vi "Filter Clusters.vi"(8 "Error In":errorcluster) -> (0 "Error Out":errorcluster)   [LabVIEW 2017]
uses:
  <vilib>/Utility/traverseref.llb/TRef TravTarget.ctl
  Support VIs/Filter Clusters Target.vi
  <vilib>/addons/_JKI Toolkits/Caraya/classes/Test/Test.lvclass
  Toolkit.lvlib
  <vilib>/Utility/traverseref.llb/VI Scripting - Traverse.lvlib
  src/Toolkit/Toolkit.lvlib
  <vilib>/addons/_JKI Toolkits/Caraya/classes/Assert/Assert.lvclass
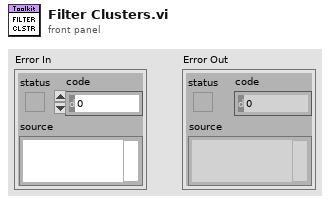
[diagram p1: front panel]
types:
  T1 = typedef "TRef TravTarget.ctl" = enum16{"FP", "BD", "Other"}
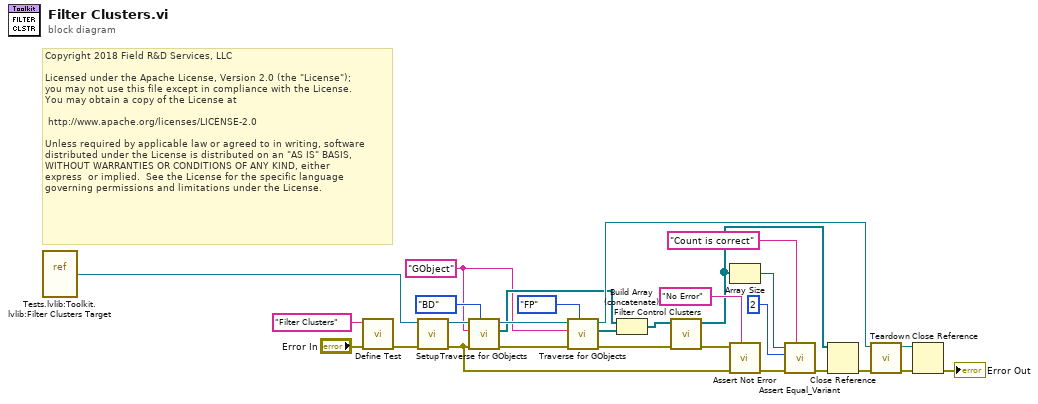
[diagram p0: block diagram]
diagram:
  w1 = "GObject" ("Class Name")
  # "Copyright 2018 Field R&D Services, LLC\n\nLicensed under the Apache License, Version 2.0 (the \"License\");\nyou may not use this file except in compliance with the License.\nYou may obtain a copy of the License at\n\n\thttp://www.apache.org/licenses/LICENSE-2.0\n\nUnless required by applicable law or agreed to in writing, software\ndistributed under the License is distributed on an \"AS IS\" BASIS,\nWITHOUT WARRANTIES OR CONDITIONS OF ANY KIND, either \nexpress  or implied.  See the License for the specific language \ngoverning permissions and limitations under the License."
  n1 = vi-ref "Tests.lvlib:Toolkit.lvlib:Filter Clusters Target.vi"() -> (w25:refnum<vi>)
  n2 = call <vilib>:"Define Test.vi"("error in (no error)"="Error In", "Label (VI Title)"="Filter Clusters") -> ("error out"=w26:errorcluster)  [unwired: 9 in]
  n3 = call "Setup.vi"("Error In"=w26, "VI In"=w25) -> ("Error Out"=w19:errorcluster, "VI Out"=w23:refnum<vi>)  [unwired: 8 in]
  n4 = call <vilib>:"Traverse for GObjects.vi"("Traverse Target"=TRef_TravTarget."BD", "error in (no error)"=w19, "Class Name"=w1, "VI Refnum"=w23) -> ("error out"=w8:errorcluster, "References"=w4:refnum<vi>[], "dup VI Refnum"=w9:refnum<vi>)  [unwired: 4 in, 1 out]
  n5 = call <vilib>:"Traverse for GObjects.vi"("Traverse Target"=TRef_TravTarget."FP", "error in (no error)"=w8, "Class Name"=w1, "VI Refnum"=w9) -> ("error out"=w7:errorcluster, "References"=w3:refnum<vi>[], "dup VI Refnum"=w6:refnum<vi>)  [unwired: 4 in, 1 out]
  n6 = Build Array (concatenate)(w4, w3) -> (w2:refnum<vi>[])
  n7 = call "Filter Control Clusters.vi"("Error In"=w7, "GObjects In"=w2) -> ("Error Out"=w20:errorcluster, "GObjects Out"=w10:refnum<vi>[])  [unwired: 8 in]
  n8 = Array Size(array=w10) -> (size(s)=w12:i32)
  n9 = call <vilib>:"Assert Not Error.vi"("Label"="No Error", "error in (no error)"=w19, "Not Error?"=w20) -> ("error out"=w14:errorcluster)  [unwired: 8 in]
  n10 = call <vilib>:"Assert Equal_Variant.vi"("Label"="Count is correct", "error in (no error)"=w14, "Y"=2 ("size(s)"), "X"=w12) -> ("error out"=w18:errorcluster)  [unwired: 7 in]
  n11 = Close Reference(reference=w10, error in (no error)=w18) -> (error out=w13:errorcluster)
  n12 = call "Teardown.vi"("Error In"=w13, "VI In"=w6) -> ("Error Out"=w16:errorcluster, "VI Out"=w17:refnum<vi>)  [unwired: 8 in]
  n13 = Close Reference(reference=w17, error in (no error)=w16) -> (error out=→"Error Out":errorcluster)
